vi "Логи_PID.vi"() -> ()   [LabVIEW 2013]
panel:
  in  "Tab Control":T1(tab)
  out "accel&gyro":cluster{dbl[], dbl[]}[](graph)
  out "uprav vosd":cluster{dbl[], dbl[]}[](graph)
  out "uprav vosd 2":cluster{dbl[], dbl[]}[](graph)
  out "Integ PID":cluster{dbl[], dbl[]}[](graph)
  out "Array 2":i16[](array[numeric])
  out "Array":i16[](array[numeric])
  out "ID параметров":u8[](array[numeric])
  out "Длина заголовка":i32
  out "Заголовок":string
  out "Количество параметров":u8
  out "size (in bytes)":i64
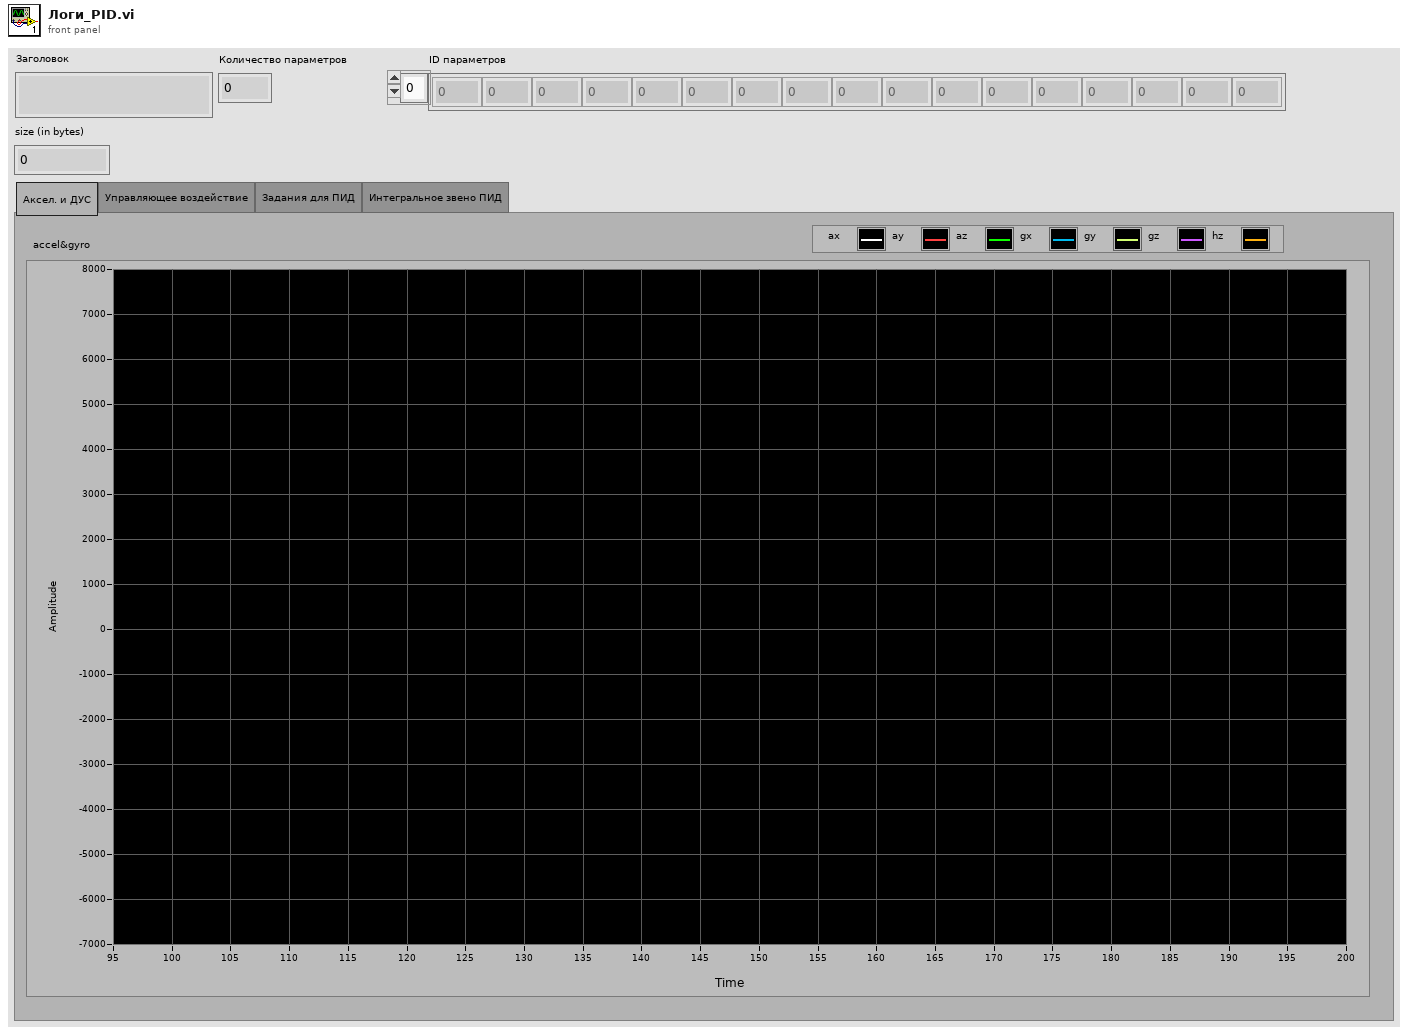
[diagram p1: front panel]
types:
  T1 = enum32{"Аксел. и ДУС", "Управляющее воздействие", "Задания для ПИД", "Интегральное звено ПИД"}
  T2 = enum16{"open", "replace", "create", "open or create", "replace or create", "replace or create with confirmation"}
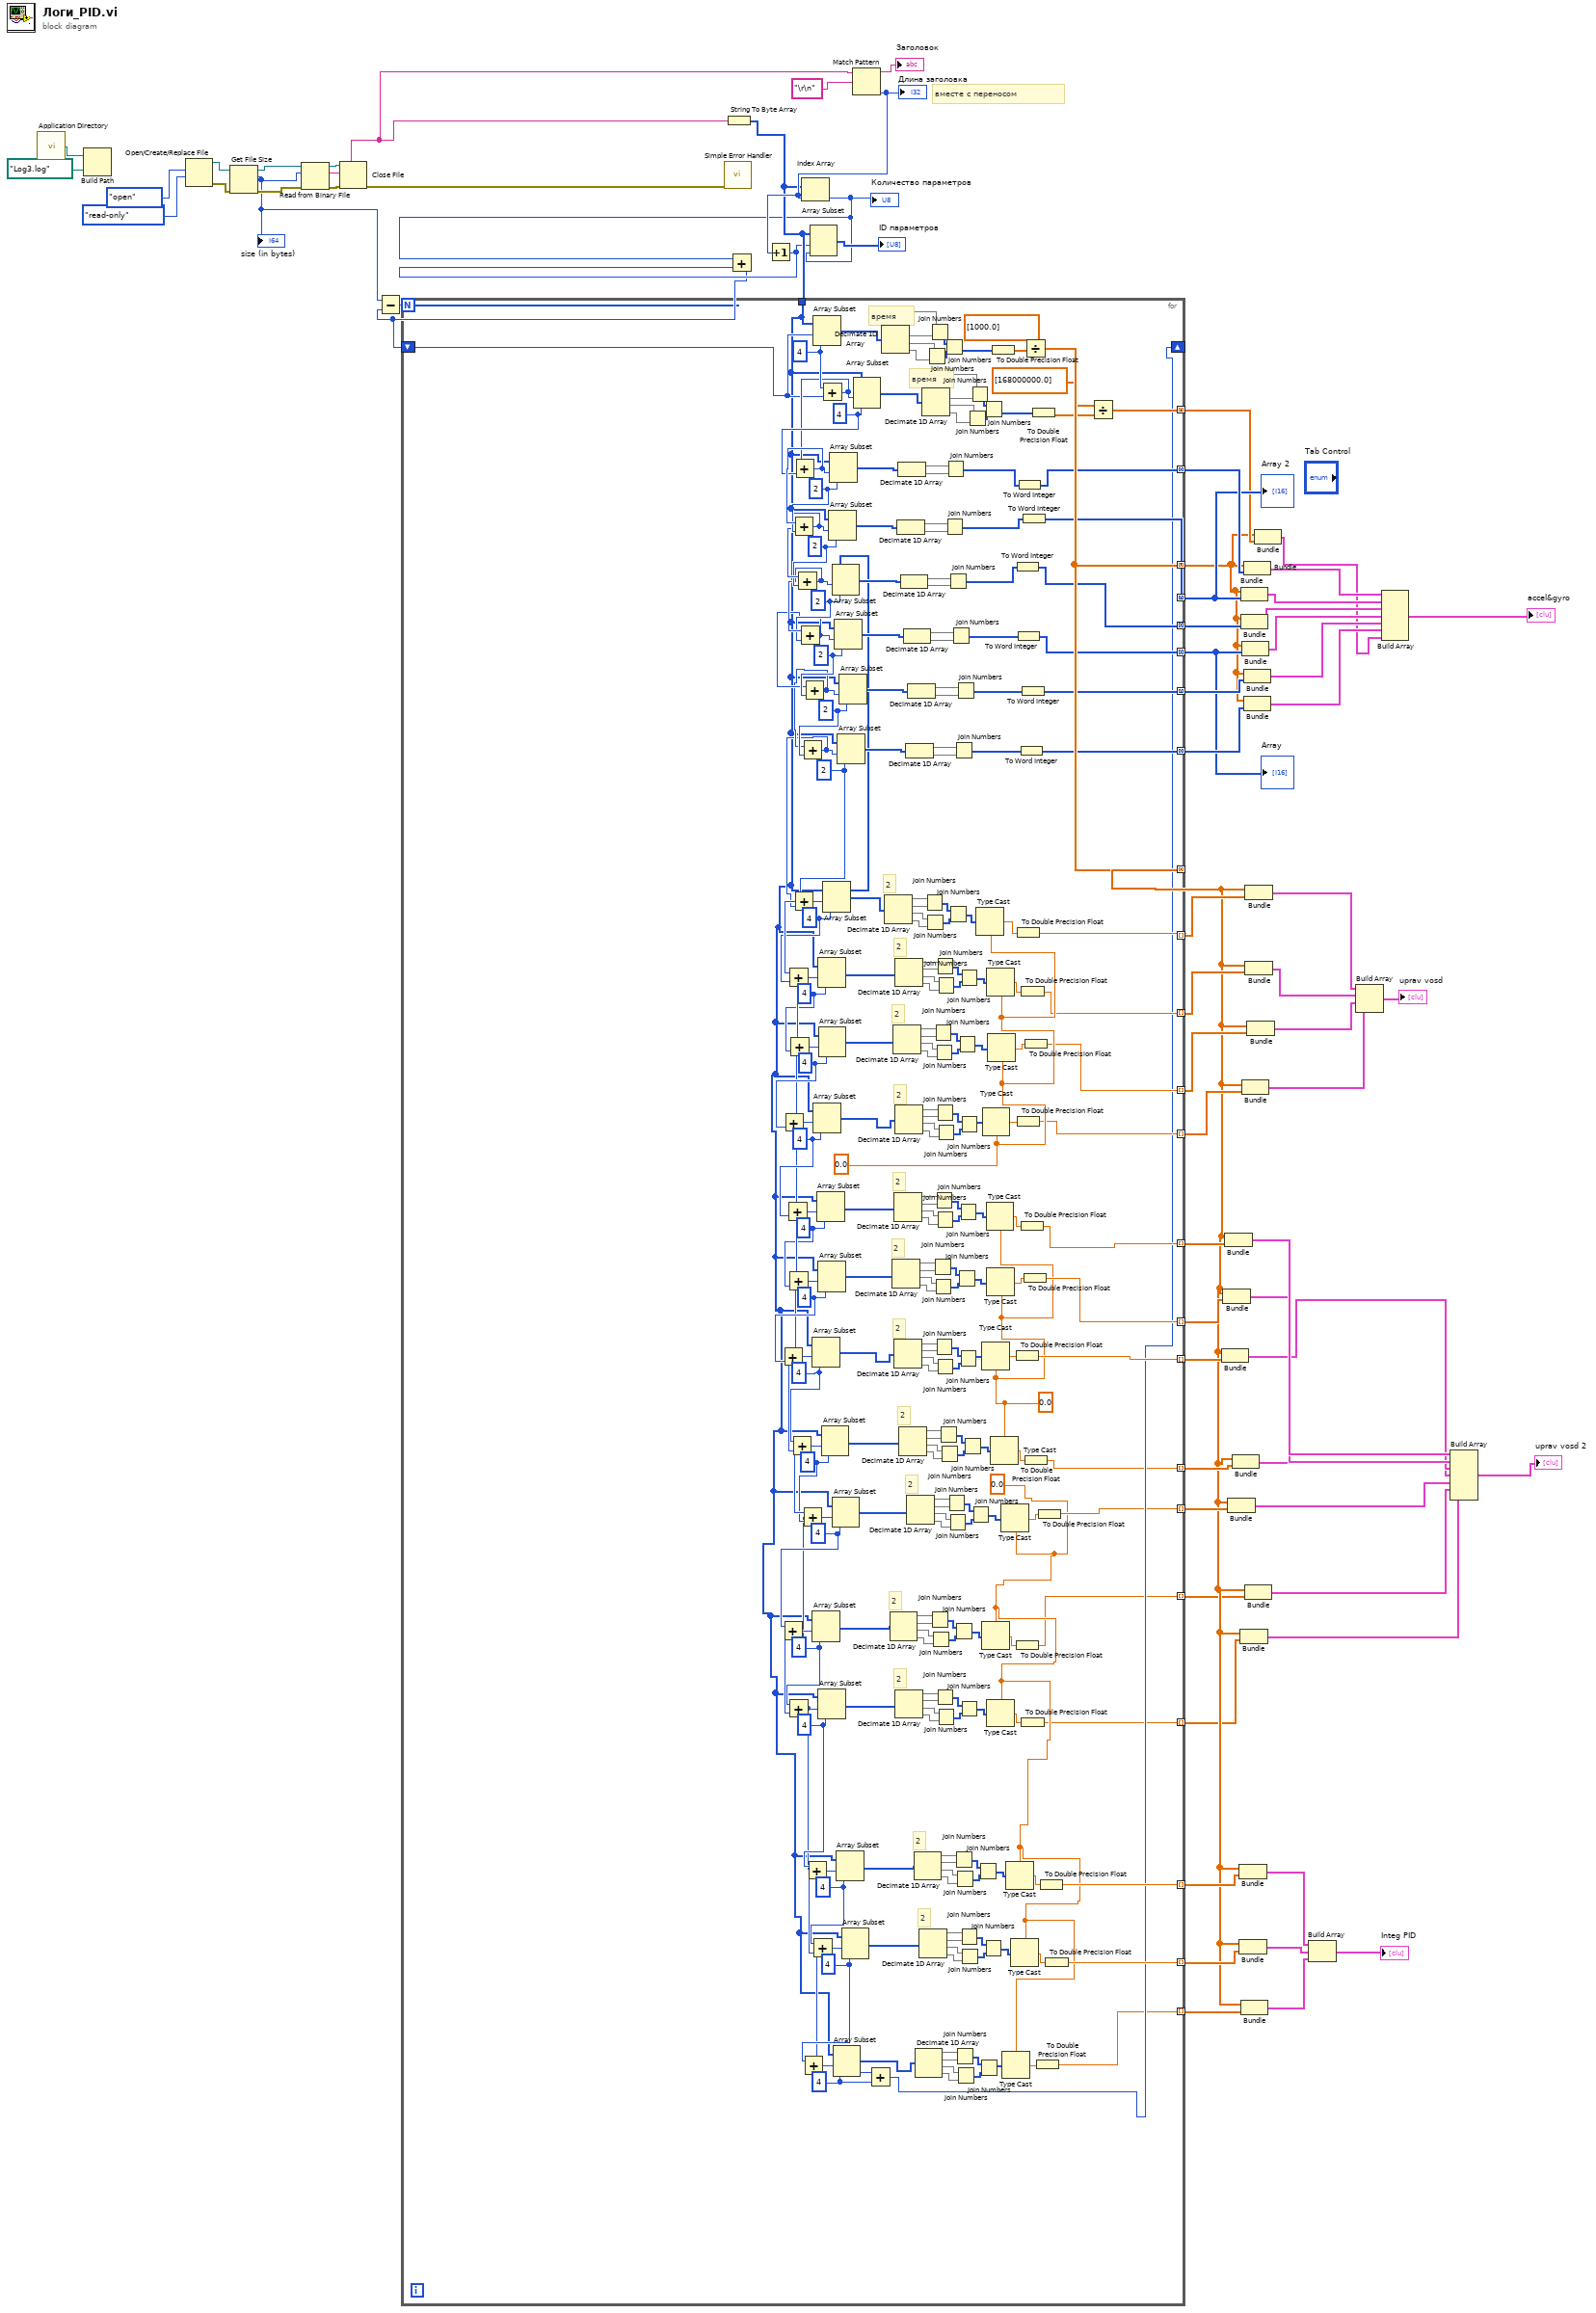
[diagram p0: block diagram]
diagram:
  # "вместе с переносом"
  n1 = call <vilib>:"Application Directory.vi"() -> ("Application Directory"=w67:path)
  n2 = Build Path(base path=w67, name or relative path=path "Log3.log" ("default name")) -> ()  [unwired: 1 out]
  n3 = Open/Create/Replace File(operation (0:open)=T2."open", access (0:read/write)=enum16{"read/write", "read-only", "write-only"}."read-only") -> (refnum out=w64:refnum<file>, error out=w62:errorcluster)  [unwired: 4 in, 1 out]
  n4 = Get File Size(file=w64, error in=w62) -> (refnum out=w63:refnum<file>, size (in bytes)=w54:i64, 0:w61:errorcluster)
  "size (in bytes)" <- w54
  n5 = Read from Binary File(8:w61, 10:w54, 11:w63) -> (0:w65:errorcluster, 2:w60:string, 3:w66:refnum<file>)  [unwired: 3 in, 1 out]
  n6 = Close File(refnum=w66, error in=w65) -> (error out=w70:errorcluster)  [unwired: 1 out]
  n7 = call <vilib>:"Simple Error Handler.vi"("error in (no error)"=w70) -> ()  [unwired: 4 in, 5 out]
  n8 = String To Byte Array(string=w60) -> (unsigned byte array=w55:u8[])
  n9 = Match Pattern(string=w60, regular expression="\r\n" ("format string")) -> (before substring=→"Заголовок":string, offset past match=w57:i32)  [unwired: 1 in, 2 out]
  "Длина заголовка" <- w57
  n10 = Increment(x=w57) -> (x+1=w52:i32)
  n11 = Index Array(array=w55, index=w57) -> (element=w53:u8)
  "Количество параметров" <- w53
  n12 = Add(x=w53, y=w52) -> (x+y=w51:i32)
  n13 = Subtract(x=w54, y=w51) -> (x-y=w50:i64)
  n14 = for {
    N: w50 -> [_]
    tunnel: w55 -> [w74]
    shift-right: [w110] -> _
    shift-left: w51 -> [w109]
    tunnel: [w240] -> w5 mode=concatenating
    tunnel: [w168] -> w17 mode=indexing
    tunnel: [w167] -> w18 mode=indexing
    tunnel: [w166] -> w19 mode=indexing
    tunnel: [w165] -> w20 mode=indexing
    tunnel: [w240] -> w28 mode=concatenating
    tunnel: [w238] -> w48 mode=concatenating
    tunnel: [w233] -> w38 mode=concatenating
    tunnel: [w235] -> w47 mode=concatenating
    tunnel: [w237] -> w36 mode=concatenating
    tunnel: [w221] -> w37 mode=concatenating
    tunnel: [w144] -> w39 mode=concatenating
    tunnel: [w185] -> w33 mode=indexing
    tunnel: [w184] -> w32 mode=indexing
    tunnel: [w183] -> w31 mode=indexing
    tunnel: [w169] -> w30 mode=concatenating
    tunnel: [w123] -> w27 mode=indexing
    tunnel: [w122] -> w26 mode=indexing
    tunnel: [w103] -> w16 mode=indexing
    tunnel: [w102] -> w13 mode=indexing
    tunnel: [w99] -> w11 mode=indexing
    tunnel: [w72] -> w4 mode=indexing
    tunnel: [w71] -> w3 mode=indexing
    w80 = 4 ("length")
    w76 = 4 ("length")
    w121 = 4 ("length")
    w125 = 4 ("length")
    w101 = 4 ("length")
    w78 = 4 ("length")
    w163 = 4 ("length")
    w73 = sgl 0.0
    w173 = 4 ("length")
    w106 = sgl 0.0
    w105 = 4 ("length")
    w218 = 4 ("length")
    w216 = 4 ("length")
    w108 = 2 ("length")
    w222 = 2 ("length")
    w223 = 2 ("length")
    w241 = 2 ("length")
    w243 = 2 ("length")
    w245 = 2 ("length")
    w261 = sgl 0.0
    w187 = 4 ("length")
    w309 = 4 ("length")
    w307 = 4 ("length")
    w310 = 4 ("length")
    w174 = 4 ("length")
    # "2"
    # "2"
    # "2"
    # "2"
    # "2"
    # "2"
    # "время"
    # "2"
    # "2"
    # "2"
    # "2"
    # "2"
    # "2"
    # "2"
    # "время"
    n15 = Array Subset(array=w74, index=w109, length=w174) -> (w296:u8[])
    n16 = Add(x=w174, y=w109) -> (x+y=w172:i32)
    n17 = Add(x=w172, y=w173) -> (x+y=w246:i32)
    n18 = Add(x=w246, y=w245) -> (x+y=w244:i32)
    n19 = Add(x=w244, y=w243) -> (x+y=w242:i32)
    n20 = Add(x=w242, y=w241) -> (x+y=w220:i32)
    n21 = Add(x=w220, y=w223) -> (x+y=w219:i32)
    n22 = Add(x=w219, y=w222) -> (x+y=w107:i32)
    n23 = Add(x=w108, y=w107) -> (x+y=w311:i32)
    n24 = Add(x=w311, y=w310) -> (x+y=w308:i32)
    n25 = Add(x=w308, y=w307) -> (x+y=w306:i32)
    n26 = Add(x=w306, y=w309) -> (x+y=w186:i32)
    n27 = Add(x=w186, y=w187) -> (x+y=w217:i32)
    n28 = Add(x=w217, y=w216) -> (x+y=w215:i32)
    n29 = Add(x=w215, y=w218) -> (x+y=w104:i32)
    n30 = Add(x=w105, y=w104) -> (x+y=w164:i32)
    n31 = Add(x=w164, y=w163) -> (x+y=w77:i32)
    n32 = Add(x=w78, y=w77) -> (x+y=w79:i32)
    n33 = Add(x=w80, y=w79) -> (x+y=w75:i32)
    n34 = Add(x=w76, y=w75) -> (x+y=w124:i32)
    n35 = Add(x=w125, y=w124) -> (x+y=w100:i32)
    n36 = Add(x=w101, y=w100) -> (x+y=w120:i32)
    n37 = Array Subset(array=w74, index=w104, length=w105) -> (w194:u8[])
    n38 = Array Subset(array=w74, index=w79, length=w80) -> (w83:u8[])
    n39 = Array Subset(array=w74, index=w186, length=w187) -> (w269:u8[])
    n40 = Array Subset(array=w74, index=w217, length=w216) -> (w208:u8[])
    n41 = Array Subset(array=w74, index=w308, length=w307) -> (w283:u8[])
    n42 = Array Subset(array=w74, index=w215, length=w218) -> (w201:u8[])
    n43 = Array Subset(array=w74, index=w75, length=w76) -> (w92:u8[])
    n44 = Array Subset(array=w74, index=w306, length=w309) -> (w276:u8[])
    n45 = Array Subset(array=w74, index=w164, length=w163) -> (w156:u8[])
    n46 = Array Subset(array=w74, index=w311, length=w310) -> (w297:u8[])
    n47 = Array Subset(array=w74, index=w244, length=w243) -> (w253:u8[])
    n48 = Array Subset(array=w74, index=w246, length=w245) -> (w256:u8[])
    n49 = Array Subset(array=w74, index=w242, length=w241) -> (w250:u8[])
    n50 = Array Subset(array=w74, index=w77, length=w78) -> (w149:u8[])
    n51 = Array Subset(array=w74, index=w120, length=w121) -> (w113:u8[])
    n52 = Array Subset(array=w74, index=w220, length=w223) -> (w247:u8[])
    n53 = Array Subset(array=w74, index=w124, length=w125) -> (w128:u8[])
    n54 = Array Subset(array=w74, index=w107, length=w108) -> (w225:u8[])
    n55 = Array Subset(array=w74, index=w219, length=w222) -> (w229:u8[])
    n56 = Array Subset(array=w74, index=w100, length=w101) -> (w137:u8[])
    n57 = Array Subset(array=w74, index=w172, length=w173) -> (w176:u8[])
    n58 = Add(x=w120, y=w121) -> (x+y=w110:i32)
    n59 = Decimate 1D Array(w296) -> (w299:u8[], w300:u8[], w301:u8[], w302:u8[])
    n60 = Decimate 1D Array(w297) -> (w304:u8[], w305:u8[], w293:u8[], w292:u8[])
    n61 = Decimate 1D Array(w83) -> (w88:u8[], w89:u8[], w87:u8[], w86:u8[])
    n62 = Decimate 1D Array(w201) -> (w206:u8[], w207:u8[], w205:u8[], w204:u8[])
    n63 = Decimate 1D Array(w276) -> (w281:u8[], w282:u8[], w280:u8[], w279:u8[])
    n64 = Decimate 1D Array(w208) -> (w213:u8[], w214:u8[], w212:u8[], w211:u8[])
    n65 = Decimate 1D Array(w194) -> (w199:u8[], w200:u8[], w198:u8[], w197:u8[])
    n66 = Decimate 1D Array(w283) -> (w288:u8[], w289:u8[], w287:u8[], w286:u8[])
    n67 = Decimate 1D Array(w269) -> (w274:u8[], w275:u8[], w273:u8[], w272:u8[])
    n68 = Decimate 1D Array(w92) -> (w97:u8[], w98:u8[], w96:u8[], w95:u8[])
    n69 = Decimate 1D Array(w253) -> (w254:u8[], w255:u8[])
    n70 = Decimate 1D Array(w256) -> (w257:u8[], w258:u8[])
    n71 = Decimate 1D Array(w156) -> (w161:u8[], w162:u8[], w160:u8[], w159:u8[])
    n72 = Decimate 1D Array(w250) -> (w251:u8[], w252:u8[])
    n73 = Decimate 1D Array(w247) -> (w248:u8[], w249:u8[])
    n74 = Decimate 1D Array(w225) -> (w226:u8[], w227:u8[])
    n75 = Decimate 1D Array(w149) -> (w154:u8[], w155:u8[], w153:u8[], w152:u8[])
    n76 = Decimate 1D Array(w229) -> (w230:u8[], w231:u8[])
    n77 = Decimate 1D Array(w128) -> (w133:u8[], w134:u8[], w132:u8[], w131:u8[])
    n78 = Decimate 1D Array(w113) -> (w118:u8[], w119:u8[], w117:u8[], w116:u8[])
    n79 = Decimate 1D Array(w137) -> (w142:u8[], w143:u8[], w141:u8[], w140:u8[])
    n80 = Join Numbers(hi=w304, lo=w305) -> ((hi.lo)=w291:u16[])
    n81 = Decimate 1D Array(w176) -> (w178:u8[], w179:u8[], w180:u8[], w181:u8[])
    n82 = Join Numbers(hi=w293, lo=w292) -> ((hi.lo)=w290:u16[])
    n83 = Join Numbers(hi=w301, lo=w302) -> ((hi.lo)=w298:u16[])
    n84 = Join Numbers(hi=w299, lo=w300) -> ((hi.lo)=w303:u16[])
    n85 = Join Numbers(hi=w88, lo=w89) -> ((hi.lo)=w85:u16[])
    n86 = Join Numbers(hi=w87, lo=w86) -> ((hi.lo)=w84:u16[])
    n87 = Join Numbers(hi=w206, lo=w207) -> ((hi.lo)=w203:u16[])
    n88 = Join Numbers(hi=w281, lo=w282) -> ((hi.lo)=w278:u16[])
    n89 = Join Numbers(hi=w205, lo=w204) -> ((hi.lo)=w202:u16[])
    n90 = Join Numbers(hi=w280, lo=w279) -> ((hi.lo)=w277:u16[])
    n91 = Join Numbers(hi=w213, lo=w214) -> ((hi.lo)=w210:u16[])
    n92 = Join Numbers(hi=w199, lo=w200) -> ((hi.lo)=w196:u16[])
    n93 = Join Numbers(hi=w288, lo=w289) -> ((hi.lo)=w285:u16[])
    n94 = Join Numbers(hi=w274, lo=w275) -> ((hi.lo)=w271:u16[])
    n95 = Join Numbers(hi=w212, lo=w211) -> ((hi.lo)=w209:u16[])
    n96 = Join Numbers(hi=w198, lo=w197) -> ((hi.lo)=w195:u16[])
    n97 = Join Numbers(hi=w97, lo=w98) -> ((hi.lo)=w94:u16[])
    n98 = Join Numbers(hi=w287, lo=w286) -> ((hi.lo)=w284:u16[])
    n99 = Join Numbers(hi=w273, lo=w272) -> ((hi.lo)=w270:u16[])
    n100 = Join Numbers(hi=w96, lo=w95) -> ((hi.lo)=w93:u16[])
    n101 = Join Numbers(hi=w161, lo=w162) -> ((hi.lo)=w158:u16[])
    n102 = Join Numbers(hi=w160, lo=w159) -> ((hi.lo)=w157:u16[])
    n103 = Join Numbers(hi=w303, lo=w298) -> ((hi.lo)=w264:u32[])
    n104 = Join Numbers(hi=w254, lo=w255) -> ((hi.lo)=w232:u16[])
    n105 = Join Numbers(hi=w257, lo=w258) -> ((hi.lo)=w239:u16[])
    n106 = Join Numbers(hi=w154, lo=w155) -> ((hi.lo)=w151:u16[])
    n107 = Join Numbers(hi=w153, lo=w152) -> ((hi.lo)=w150:u16[])
    n108 = Join Numbers(hi=w251, lo=w252) -> ((hi.lo)=w234:u16[])
    n109 = Join Numbers(hi=w291, lo=w290) -> ((hi.lo)=w260:u32[])
    n110 = Join Numbers(hi=w248, lo=w249) -> ((hi.lo)=w236:u16[])
    n111 = Join Numbers(hi=w226, lo=w227) -> ((hi.lo)=w224:u16[])
    n112 = Join Numbers(hi=w85, lo=w84) -> ((hi.lo)=w82:u32[])
    n113 = Join Numbers(hi=w133, lo=w134) -> ((hi.lo)=w130:u16[])
    n114 = Join Numbers(hi=w132, lo=w131) -> ((hi.lo)=w129:u16[])
    n115 = Join Numbers(hi=w118, lo=w119) -> ((hi.lo)=w115:u16[])
    n116 = Join Numbers(hi=w230, lo=w231) -> ((hi.lo)=w228:u16[])
    n117 = Join Numbers(hi=w117, lo=w116) -> ((hi.lo)=w114:u16[])
    n118 = Join Numbers(hi=w203, lo=w202) -> ((hi.lo)=w191:u32[])
    n119 = Join Numbers(hi=w278, lo=w277) -> ((hi.lo)=w266:u32[])
    n120 = Join Numbers(hi=w210, lo=w209) -> ((hi.lo)=w189:u32[])
    n121 = Join Numbers(hi=w196, lo=w195) -> ((hi.lo)=w192:u32[])
    n122 = Join Numbers(hi=w285, lo=w284) -> ((hi.lo)=w263:u32[])
    n123 = Join Numbers(hi=w271, lo=w270) -> ((hi.lo)=w267:u32[])
    n124 = Join Numbers(hi=w94, lo=w93) -> ((hi.lo)=w91:u32[])
    n125 = Join Numbers(hi=w142, lo=w143) -> ((hi.lo)=w139:u16[])
    n126 = Join Numbers(hi=w141, lo=w140) -> ((hi.lo)=w138:u16[])
    n127 = Join Numbers(hi=w158, lo=w157) -> ((hi.lo)=w146:u32[])
    n128 = Join Numbers(hi=w180, lo=w181) -> ((hi.lo)=w177:u16[])
    n129 = Join Numbers(hi=w178, lo=w179) -> ((hi.lo)=w182:u16[])
    n130 = Join Numbers(hi=w151, lo=w150) -> ((hi.lo)=w148:u32[])
    n131 = Join Numbers(hi=w130, lo=w129) -> ((hi.lo)=w127:u32[])
    n132 = Join Numbers(hi=w115, lo=w114) -> ((hi.lo)=w111:u32[])
    n133 = Type Cast(type=w261, x=w260) -> (*(type *) &x=w259:sgl)
    n134 = Join Numbers(hi=w139, lo=w138) -> ((hi.lo)=w136:u32[])
    n135 = Join Numbers(hi=w182, lo=w177) -> ((hi.lo)=w175:u32[])
    n136 = Type Cast(type=w106, x=w192) -> (*(type *) &x=w193:sgl)
    n137 = Type Cast(type=w73, x=w82) -> (*(type *) &x=w81:sgl)
    n138 = Type Cast(type=w261, x=w267) -> (*(type *) &x=w268:sgl)
    n139 = Type Cast(type=w106, x=w189) -> (*(type *) &x=w188:sgl)
    n140 = Type Cast(type=w261, x=w263) -> (*(type *) &x=w262:sgl)
    n141 = Type Cast(type=w106, x=w191) -> (*(type *) &x=w190:sgl)
    n142 = Type Cast(type=w73, x=w91) -> (*(type *) &x=w90:sgl)
    n143 = Type Cast(type=w261, x=w266) -> (*(type *) &x=w265:sgl)
    n144 = To Double Precision Float(number=w264) -> (double precision float=w295:dbl[])
    n145 = Type Cast(type=w106, x=w146) -> (*(type *) &x=w145:sgl)
    n146 = Type Cast(type=w73, x=w148) -> (*(type *) &x=w147:sgl)
    n147 = Type Cast(type=w73, x=w111) -> (*(type *) &x=w112:sgl)
    n148 = Type Cast(type=w73, x=w127) -> (*(type *) &x=w126:sgl)
    n149 = Type Cast(type=w73, x=w136) -> (*(type *) &x=w135:sgl)
    n150 = To Word Integer(number=w234) -> (16bit integer=w235:i16[])
    n151 = To Double Precision Float(number=w193) -> (double precision float=w183:dbl)
    n152 = To Double Precision Float(number=w81) -> (double precision float=w72:dbl)
    n153 = To Word Integer(number=w236) -> (16bit integer=w237:i16[])
    n154 = To Double Precision Float(number=w259) -> (double precision float=w168:dbl)
    n155 = To Double Precision Float(number=w268) -> (double precision float=w165:dbl)
    n156 = To Word Integer(number=w239) -> (16bit integer=w238:i16[])
    n157 = To Word Integer(number=w224) -> (16bit integer=w144:i16[])
    n158 = To Double Precision Float(number=w188) -> (double precision float=w185:dbl)
    n159 = To Word Integer(number=w228) -> (16bit integer=w221:i16[])
    n160 = To Double Precision Float(number=w262) -> (double precision float=w167:dbl)
    n161 = To Double Precision Float(number=w90) -> (double precision float=w71:dbl)
    n162 = To Word Integer(number=w232) -> (16bit integer=w233:i16[])
    n163 = Divide(x=w295, y=dbl[] [1000.0]) -> (x/y=w240:dbl[])
    n164 = To Double Precision Float(number=w190) -> (double precision float=w184:dbl)
    n165 = To Double Precision Float(number=w265) -> (double precision float=w166:dbl)
    n166 = To Double Precision Float(number=w145) -> (double precision float=w103:dbl)
    n167 = To Double Precision Float(number=w175) -> (double precision float=w171:dbl[])
    n168 = To Double Precision Float(number=w112) -> (double precision float=w99:dbl)
    n169 = To Double Precision Float(number=w147) -> (double precision float=w102:dbl)
    n170 = To Double Precision Float(number=w126) -> (double precision float=w123:dbl)
    n171 = To Double Precision Float(number=w135) -> (double precision float=w122:dbl)
    n172 = Divide(x=dbl[] [168000000.0] ("y"), y=w171) -> (x/y=w169:dbl[])
  }
  "Array" <- w36
  "Array 2" <- w38
  n173 = Array Subset(array=w55, index=w52, length=w53) -> (→"ID параметров":u8[])
  n174 = Bundle(w5, w31) -> (w15:cluster{dbl[], dbl[]})  [unwired: 1 in]
  n175 = Bundle(w5, w32) -> (w34:cluster{dbl[], dbl[]})  [unwired: 1 in]
  n176 = Bundle(w5, w33) -> (w35:cluster{dbl[], dbl[]})  [unwired: 1 in]
  n177 = Bundle(w5, w13) -> (w12:cluster{dbl[], dbl[]})  [unwired: 1 in]
  n178 = Bundle(w5, w16) -> (w14:cluster{dbl[], dbl[]})  [unwired: 1 in]
  n179 = Bundle(w5, w27) -> (w10:cluster{dbl[], dbl[]})  [unwired: 1 in]
  n180 = Bundle(w5, w26) -> (w9:cluster{dbl[], dbl[]})  [unwired: 1 in]
  n181 = Bundle(w5, w3) -> (w1:cluster{dbl[], dbl[]})  [unwired: 1 in]
  n182 = Bundle(w28, w38) -> (w45:cluster{dbl[], i16[]})  [unwired: 1 in]
  n183 = Bundle(w28, w47) -> (w44:cluster{dbl[], i16[]})  [unwired: 1 in]
  n184 = Bundle(w5, w11) -> (w8:cluster{dbl[], dbl[]})  [unwired: 1 in]
  n185 = Bundle(w28, w36) -> (w43:cluster{dbl[], i16[]})  [unwired: 1 in]
  n186 = Bundle(w5, w20) -> (w22:cluster{dbl[], dbl[]})  [unwired: 1 in]
  n187 = Bundle(w28, w48) -> (w46:cluster{dbl[], i16[]})  [unwired: 1 in]
  n188 = Bundle(w28, w37) -> (w41:cluster{dbl[], i16[]})  [unwired: 1 in]
  n189 = Bundle(w28, w39) -> (w40:cluster{dbl[], i16[]})  [unwired: 1 in]
  n190 = Bundle(w5, w4) -> (w2:cluster{dbl[], dbl[]})  [unwired: 1 in]
  n191 = Bundle(w5, w17) -> (w25:cluster{dbl[], dbl[]})  [unwired: 1 in]
  n192 = Bundle(w5, w18) -> (w24:cluster{dbl[], dbl[]})  [unwired: 1 in]
  n193 = Bundle(w5, w19) -> (w23:cluster{dbl[], dbl[]})  [unwired: 1 in]
  n194 = Bundle(w28, w30) -> (w29:cluster{dbl[], dbl[]})  [unwired: 1 in]
  n195 = Build Array(w10, w9, w8) -> (→"Integ PID":cluster{dbl[], dbl[]}[])
  n196 = Build Array(w25, w24, w23, w22) -> (→"uprav vosd":cluster{dbl[], dbl[]}[])
  n197 = Build Array(w46, w45, w44, w43, w41, w40, w29) -> (→"accel&gyro":cluster{dbl[], dbl[]}[])
  n198 = Build Array(w35, w34, w15, w14, w12, w2, w1) -> (→"uprav vosd 2":cluster{dbl[], dbl[]}[])
